vi "Cleanup.vi"(0 "Operation Interface in":refnum<class "Operation Interface.lvclass">) -> ()   [LabVIEW 2016, in "Operation Interface.lvclass"]
uses:
  Operation Interface.lvclass
  Operation Interface.lvclass/Operation Interface.ctl
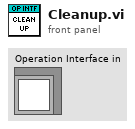
[diagram p1: front panel]
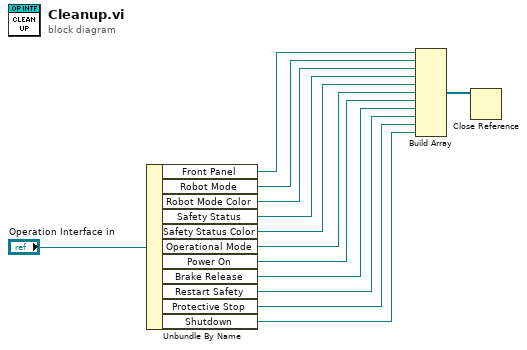
[diagram p0: block diagram]
diagram:
  n1 = Unbundle By Name("Operation Interface in") -> ("Front Panel"=w12:refnum<vi>, "Robot Mode"=w11:refnum<vi>, "Robot Mode Color"=w10:refnum<vi>, "Safety Status"=w9:refnum<vi>, "Safety Status Color"=w8:refnum<vi>, "Operational Mode"=w7:refnum<vi>, "Power On"=w6:refnum<vi>, "Brake Release"=w5:refnum<vi>, "Restart Safety"=w4:refnum<vi>, "Protective Stop"=w3:refnum<vi>, "Shutdown"=w2:refnum<vi>)
  n2 = Build Array(w12, w11, w10, w9, w8, w7, w6, w5, w4, w3, w2) -> (w1:refnum<vi>[])
  n3 = Close Reference(reference=w1) -> ()  [unwired: 1 in, 1 out]
